vi "DATA MONITOR .vi"() -> ()   [LabVIEW 2018]
uses:
  <vilib>/Utility/miscctls.llb/LVRectTypeDef.ctl
panel:
  out "Date":string
  out "Year":string
  in  "Offset 7":u16 caption="Gain" max=100 format="%.0f "
  in  "Gain 7":u16 caption="Gain" max=100 format="%.0f "
  in  "Offset 5":u16 caption="Gain" max=100 format="%.0f "
  in  "Gain 5":u16 caption="Gain" max=100 format="%.0f "
  in  "Offset 6":u16 caption="Gain" max=100 format="%.0f "
  in  "Gain 6":u16 caption="Gain" max=100 format="%.0f "
  in  "Offset 3":u16 caption="Gain" max=100 format="%.0f "
  in  "Gain 3":u16 caption="Gain" max=100 format="%.0f "
  in  "Offset 4":u16 caption="Gain" max=100 format="%.0f "
  in  "Gain 4":u16 caption="Gain" max=100 format="%.0f "
  in  "Offset 1":u16 caption="Gain" max=100 format="%.0f "
  in  "Gain  1":u16 caption="Gain" max=100 format="%.0f "
  in  "Offset 2":u16 caption="Gain" max=100 format="%.0f "
  in  "Gain  2":u16 caption="Gain" max=100 format="%.0f "
  in  "Safety Limits":bool
  out "Dynamometer Torque N-m 8":dbl(knob) caption="Basement_T" scale=0.0..100.0
  out "Temperature PID":bool
  in  "Temperature":dbl(slide) scale=0.0..10.0
  out "Eng Rpm 2":dbl(knob) caption="Power" scale=0.0..10000.0
  out "Eng Rpm":dbl(knob) caption="Torque Summary" scale=0.0..10000.0
  out "Dynorpm":dbl(knob) caption="Speed Summary" scale=0.0..8000.0
  out "Dynamometer Torque N-m 7":dbl(knob) caption="Coolant_Outlet_T" scale=0.0..100.0
  out "Dynamometer Torque N-m 6":dbl(knob) caption="Coolant_Inlet_T" scale=0.0..100.0
  out "Dynamometer Torque N-m 5":dbl(knob) caption="Exhaust_T" scale=0.0..100.0
  out "Dynamometer Torque N-m 4":dbl(knob) caption="Oil_T" scale=0.0..100.0
  out "Dynamometer Torque N-m 3":dbl(knob) caption="Intercooler_Out_T" scale=0.0..100.0
  out "Dynamometer Torque N-m 2":dbl(knob) caption="Intercooler_In_T" scale=0.0..100.0
  in  "Reset":bool
  out "Alarms & Status":string
  in  "Tab Control":enum32{"Pressure  parameter", "Graph"}(tab)
  out "Ambient Temp. 2":dbl(slide) caption="Intercooler-In_P" scale=0.0..200.0
  out "Spark plug Temp":dbl(slide) caption="Coolant-Out_P" scale=0.0..200.0
  out "Oil Temp.":dbl(slide) caption="Coolant-In_P" scale=0.0..120.0
  out "Cylinder Block Temp.":dbl(slide) caption="Exhaust_P" scale=0.0..120.0
  out "ExhaustTemp.":dbl(slide) caption="Oil_P" scale=0.0..200.0
  out "Ambient Temp.":dbl(slide) caption="Intercooler-Out_P" scale=0.0..200.0
  out "T1":dbl(slide) caption="Misc_P" scale=0.0..100.0
  out "Chart 2":i32[](graph)
  out "eng model":string caption="Engine Model"
  out "eng type":string caption="Engine Type"
  out "NI cRIO Comm.":bool
  out "Test Cycle":dbl format="%<%H:%M:%S>t"
  in  "test stop":bool
  in  "start":bool
  in  "Home Button":bool
  # "ONLINE DATA"
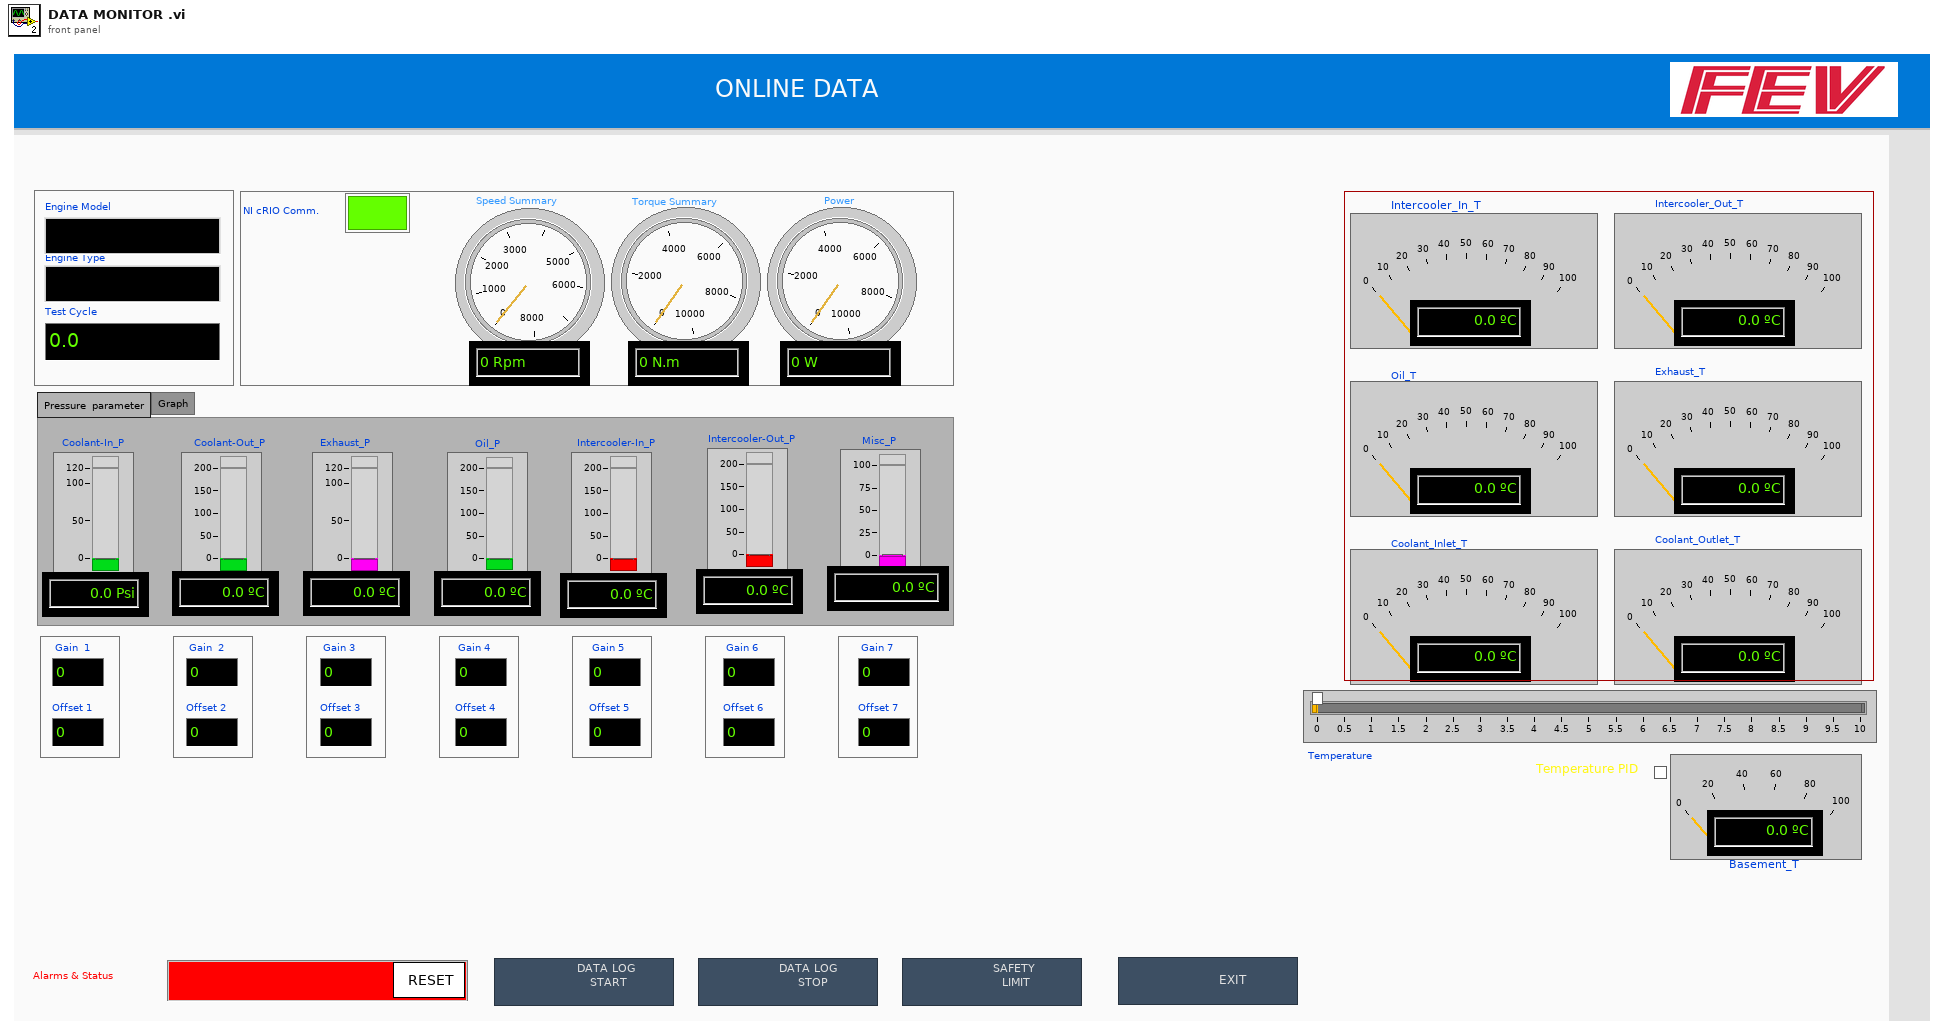
[diagram p1: front panel]
types:
  T1 = enum32{"Invalid", "Standard", "Closed", "Hidden", "Minimized", "Maximized"}
  T2 = enum32{"invalid app kind", "Development System", "Run Time System", "Student Edition", "Embedded LabVIEW", "Evaluation", "Custom"}
  T3 = typedef "LVRectTypeDef.ctl" = cluster{"Left":i16, "Top":i16, "Right":i16, "Bottom":i16}
  T4 = cluster{"Core":cluster{"Current VI Reference":refnum<vi>, "Close Panel on Exit?":bool}, "Your Boolean data":bool, "Your string data":string}
  T5 = cluster{"Current VI Reference":refnum<vi>, "Close Panel on Exit?":bool}
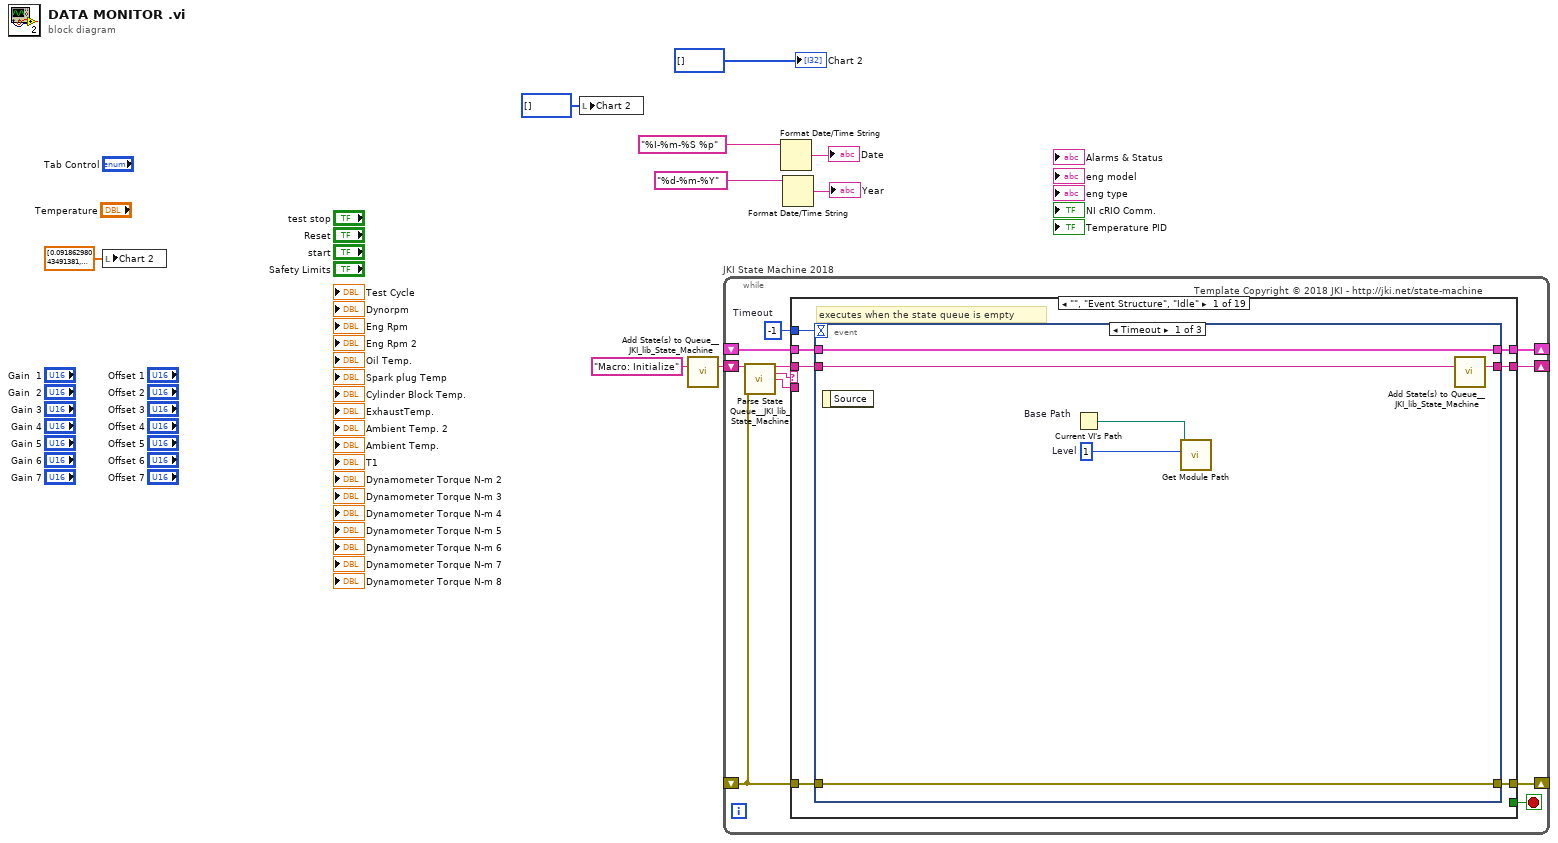
[diagram p0: block diagram]
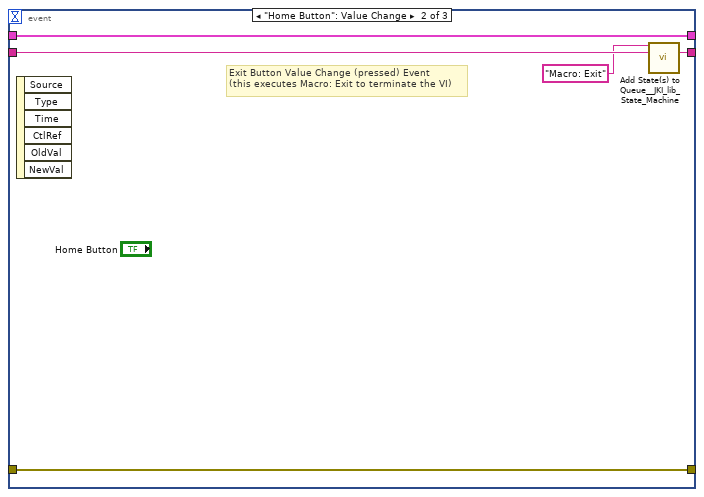
[diagram p2: hidden frame]
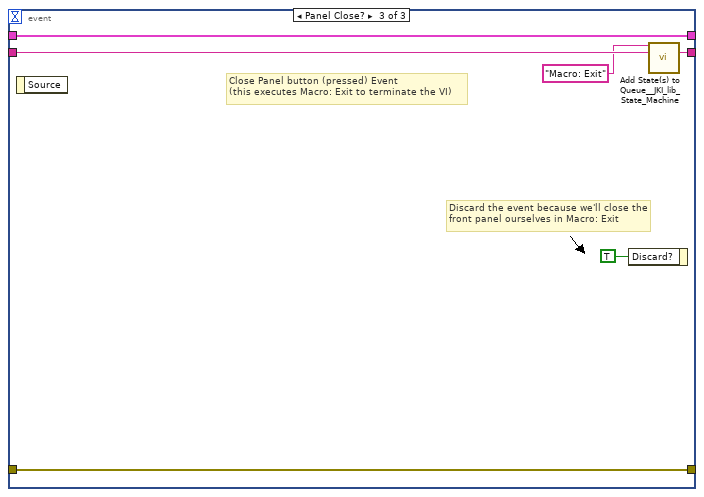
[diagram p3: hidden frame]
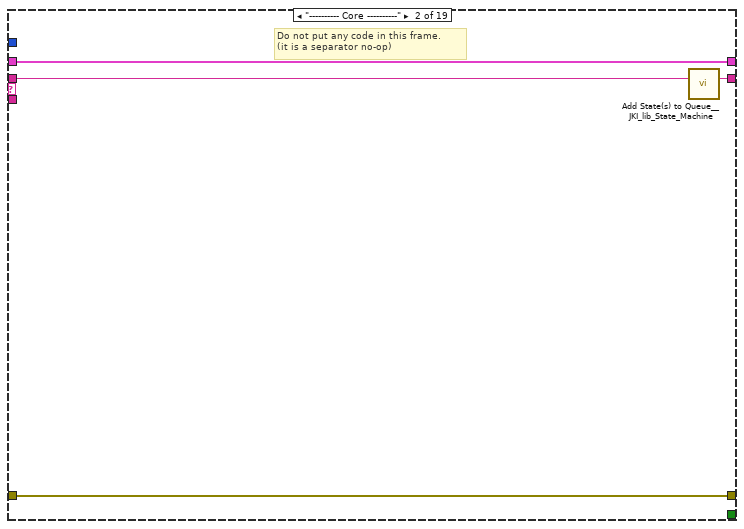
[diagram p4: hidden frame]
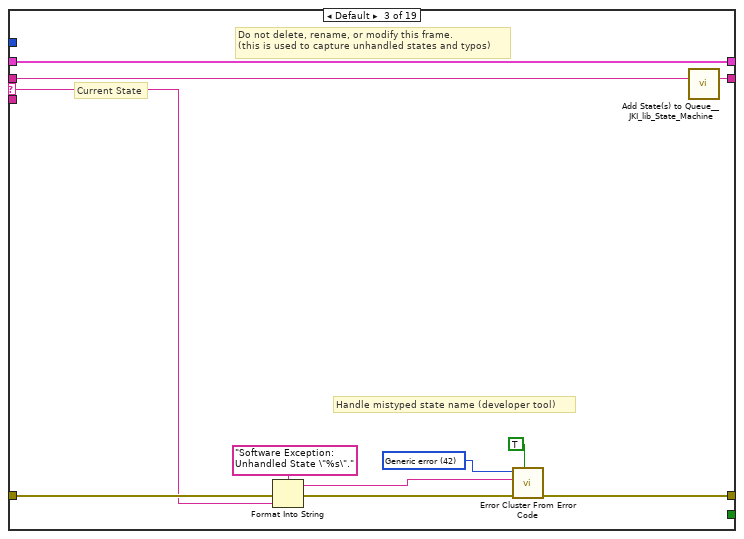
[diagram p5: hidden frame]
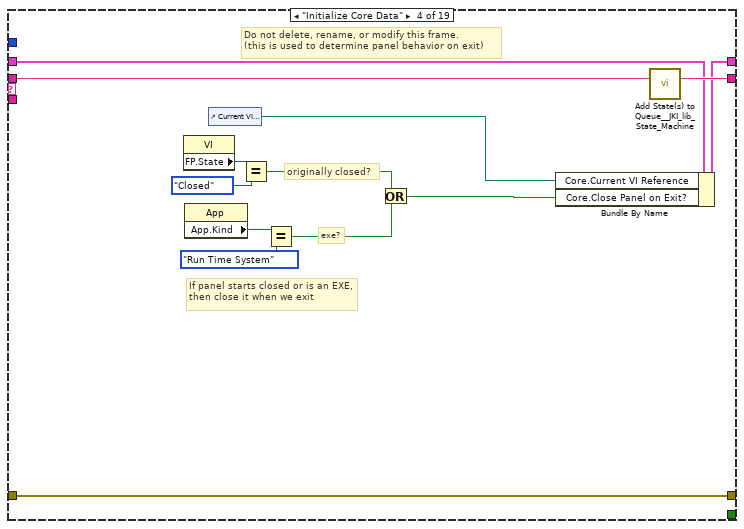
[diagram p6: hidden frame]
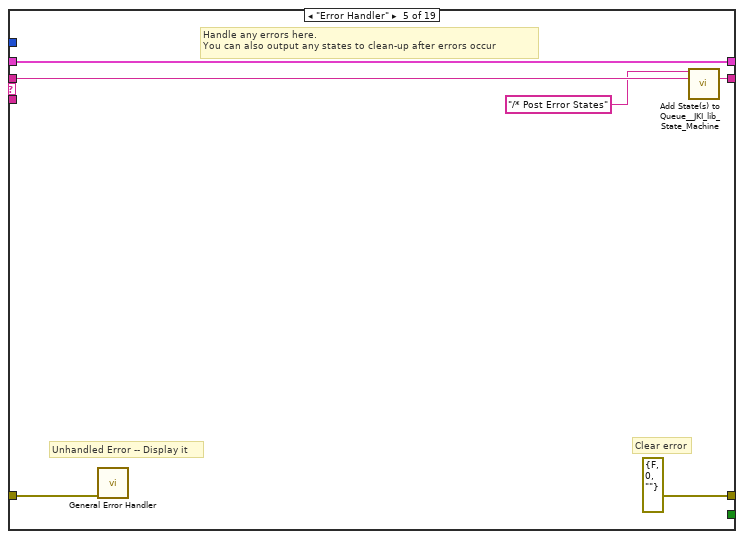
[diagram p7: hidden frame]
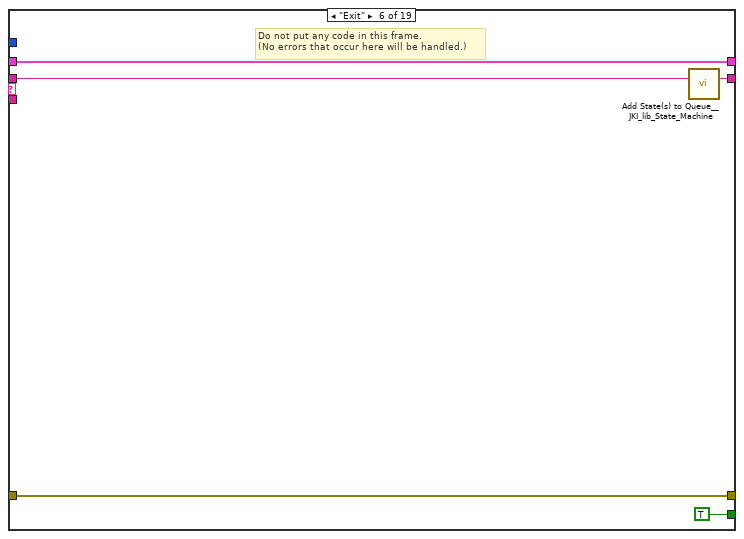
[diagram p8: hidden frame]
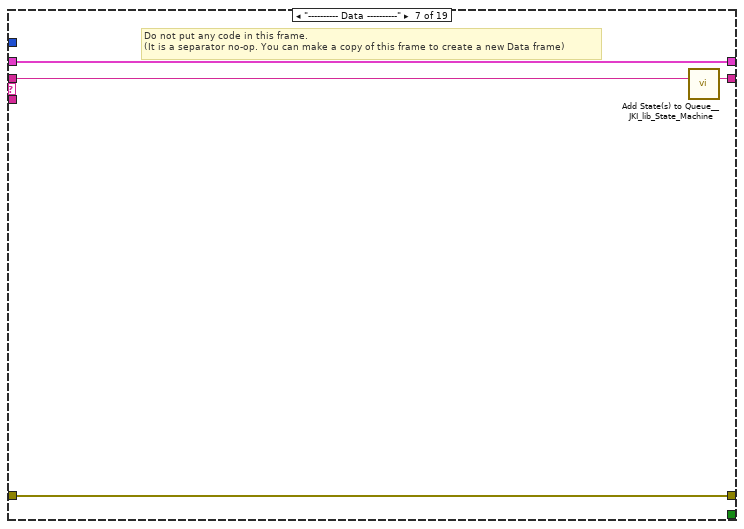
[diagram p9: hidden frame]
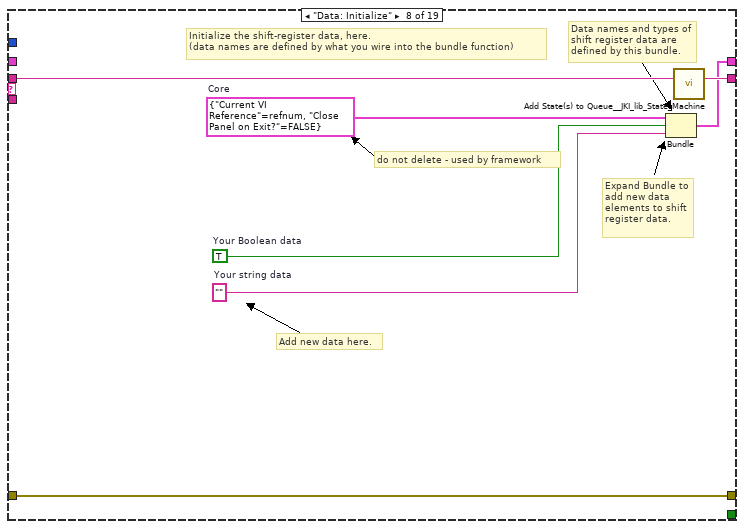
[diagram p10: hidden frame]
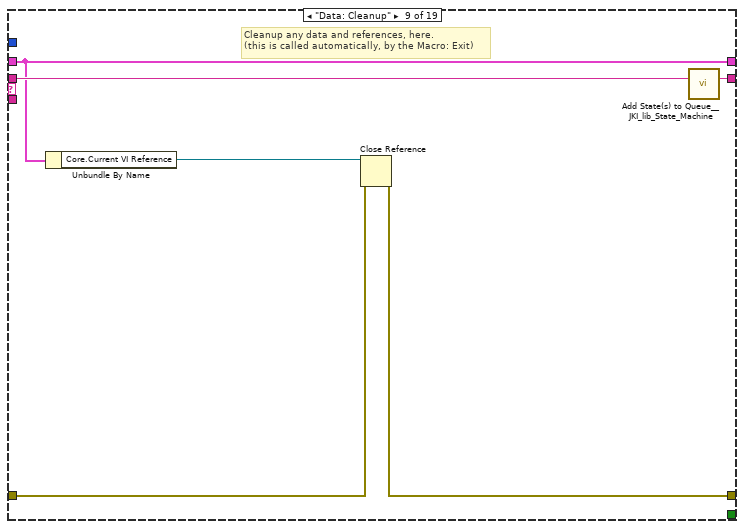
[diagram p11: hidden frame]
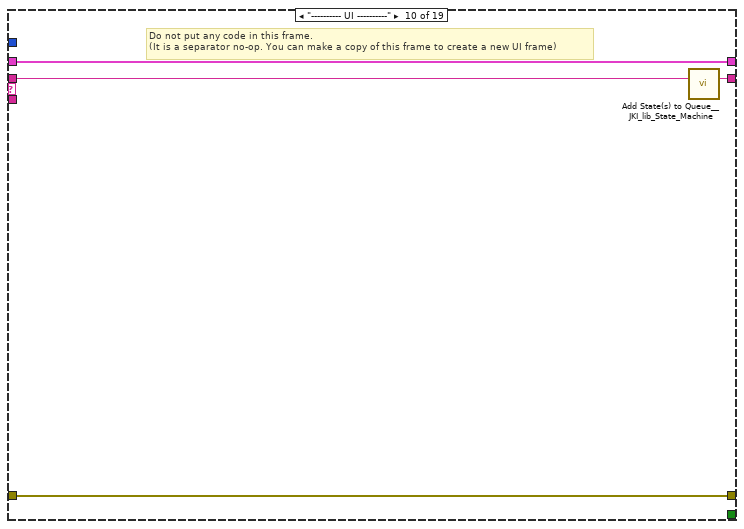
[diagram p12: hidden frame]
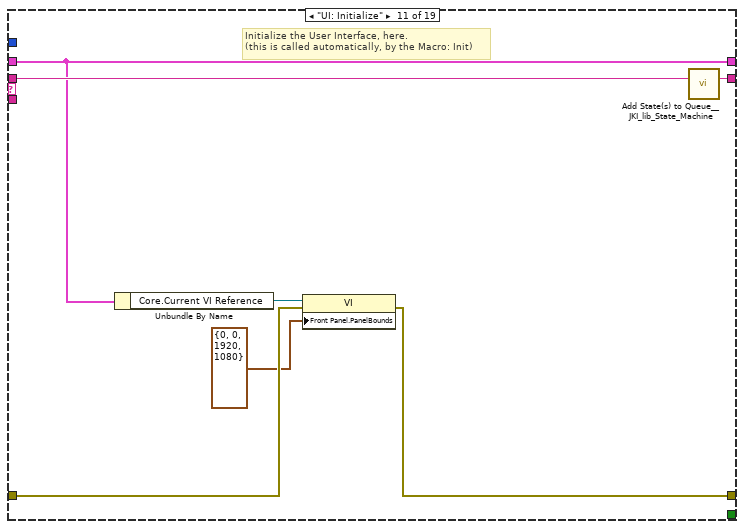
[diagram p13: hidden frame]
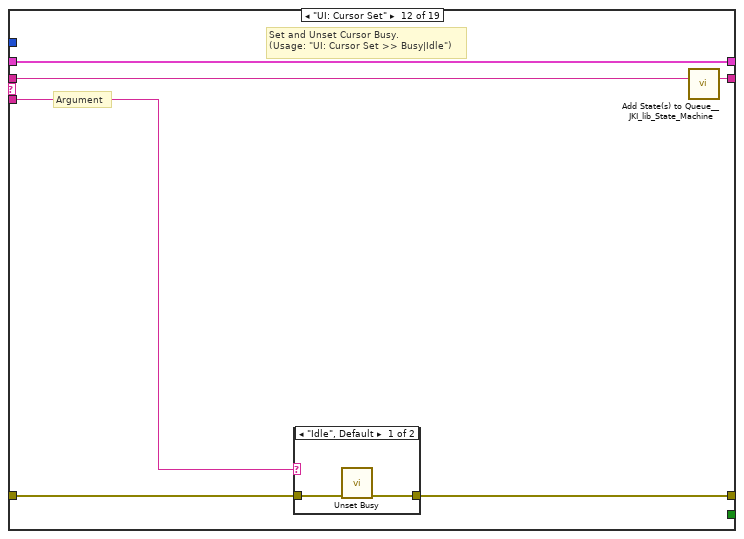
[diagram p14: hidden frame]
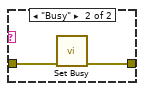
[diagram p15: hidden frame]
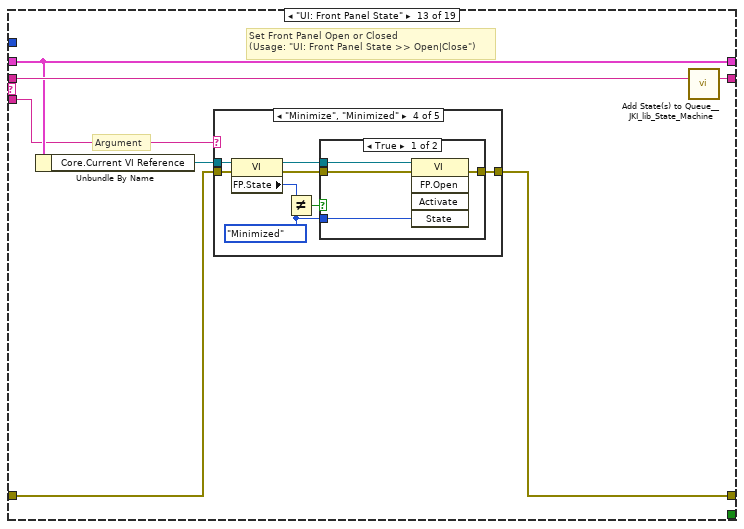
[diagram p16: hidden frame]
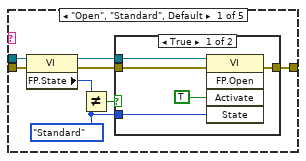
[diagram p17: hidden frame]
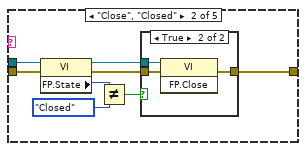
[diagram p19: hidden frame]
diagram:
  n1 = local write "Chart 2"(dbl[] [0.09186298043491381, 5.091862980434914, 0.09186298043491381] ("Chart 2")) -> ()
  n2 = local write "Chart 2"(i32[] [] ("Chart 2")) -> ()
  n3 = call <vilib>:"Add State(s) to Queue__JKI_lib_State_Machine.vi"("State(s) in (\"\")"="Macro: Initialize") -> ("States Out"=w2:string)  [unwired: 14 in]
  n4 = while "JKI State Machine 2018" {
    shift-right: [w13] -> _
    shift-left: _ -> [w12]
    shift-right: [w16] -> _
    shift-left: _ -> [w10]
    shift-right: [w15] -> _
    shift-left: w2 -> [w17]
    stop <- w14 stop-if-true
    w11 = -1  # Timeout
    # "Template Copyright © 2018 JKI - http://jki.net/state-machine"
    n5 = call <vilib>:"Parse State Queue__JKI_lib_State_Machine.vi"("State Queue"=w17, "Error In (no error)"=w10) -> ("Remaining States"=w19:string, "Current State"=w20:string, "Arguments"=w18:string)  [unwired: 11 in]
    n6 = case shown="\"\", \"Event Structure\", \"Idle\"" w20 {
      selector: w20 -> [_ _ w49 _ _ _ _ _ _ _ _ _ _ _ _ _ _ _ _]
      tunnel: w19 -> [w27 w48 w53 w72 w78 w83 w87 w94 w100 w104 w111 w117 w128 w197 w202 w212 w216 w220 w224]
      tunnel: w18 -> [_ _ _ _ _ _ _ _ _ _ _ w112 w122 _ _ _ _ _ _]
      tunnel: w12 -> [w25 w45 w51 w65 w75 w81 w84 _ w95 w101 w109 w115 w124 w194 w199 w209 w213 w217 w221]
      tunnel: [w24 w46 w55 w69 errorcluster {"status"=FALSE, "code"=0, "source"=""} ("error out") w80 w85 w91 w96 w102 w106 w113 w125 w195 w200 w210 w214 w218 w222] -> w16
      tunnel: w10 -> [w23 w46 w54 w69 w74 w80 w85 w91 w97 w102 w107 w114 w126 w195 w200 w210 w214 w218 w222]
      tunnel: [w26 w47 w52 w71 w77 w82 w86 w93 w99 w103 w110 w116 w127 w196 w201 w211 w215 w219 w223] -> w15
      tunnel: [_ _ _ _ _ TRUE _ _ _ _ _ _ _ _ _ _ _ _ _] -> w14
      tunnel: [w22 w45 w51 w70 w75 w81 w84 w92 w95 w101 w109 w115 w124 w194 w199 w209 w213 w217 w221] -> w13
      tunnel: w11 -> [w21 _ _ _ _ _ _ _ _ _ _ _ _ _ _ _ _ _ _]
      frame "", "Event Structure", "Idle" {
        # "executes when the state queue is empty"
        n7 = event shown="[0] Timeout" {
          selector: _ -> [_ _ _]
          dyn-events: _ -> [_ _ _]
          timeout: w21 -> [_ _ _]
          tunnel: w27 -> [w33 w38 w44]
          tunnel: [w32 w37 w43] -> w26
          tunnel: w25 -> [w30 w35 w41]
          tunnel: [w31 w36 w42] -> w24
          tunnel: w23 -> [w31 w36 w42]
          tunnel: [w30 w35 w41] -> w22
          event Timeout {
            w28 = 1  # Level
            n8 = event-data() -> ()  [unwired: 1 in, 1 out]
            n9 = Current VI's Path "Base Path"() -> (path=w29:path)
            n10 = call "Get Module Path.vi"("Level"=w28, "path"=w29) -> ()  [unwired: 8 in, 2 out]
            n11 = call <vilib>:"Add State(s) to Queue__JKI_lib_State_Machine.vi"("State(s) in (\"\")"=w33) -> ("States Out"=w32:string)  [unwired: 14 in]
          }
          event "Home Button": Value Change {
            # "Exit Button Value Change (pressed) Event\n(this executes Macro: Exit to terminate the VI)"
            n12 = event-data() -> ()  [unwired: 1 in, 6 out]
            n13 = call <vilib>:"Add State(s) to Queue__JKI_lib_State_Machine.vi"("State(s) in Front (\"\")"="Macro: Exit", "State(s) in (\"\")"=w38) -> ("States Out"=w37:string)  [unwired: 13 in]
          }
          event Panel Close? {
            # "Discard the event because we'll close the front panel ourselves in Macro: Exit"
            # "Close Panel button (pressed) Event\n(this executes Macro: Exit to terminate the VI)"
            n14 = event-data() -> ()  [unwired: 1 in, 1 out]
            n15 = event-data("Discard?"=TRUE) -> ()  [unwired: 1 in, 1 out]
            n16 = call <vilib>:"Add State(s) to Queue__JKI_lib_State_Machine.vi"("State(s) in Front (\"\")"="Macro: Exit", "State(s) in (\"\")"=w44) -> ("States Out"=w43:string)  [unwired: 13 in]
          }
        }
      }
      frame "---------- Core ----------" {
        # "Do not put any code in this frame.\n(it is a separator no-op)"
        n17 = call <vilib>:"Add State(s) to Queue__JKI_lib_State_Machine.vi"("State(s) in (\"\")"=w48) -> ("States Out"=w47:string)  [unwired: 14 in]
      }
      frame Default {
        w58 = 42 items=["No error", "Argument error", "Memory is full", "Out of zone", "End of file", "File already open", "Generic file I/O error", "File not found", "File permission error", "Disk is full", "Duplicate path", "Too many files open", "System feature not enabled", "Resource file not found", "Cannot add resource", "Resource not found", "Image not found", "Image memory error", "Pen does not exist", "Config type invalid", "Config token not found", "Config parse error", "Config memory error", "Bad external code format", "Bad external code offset", "External code not present", "Null window", "Destroy window error", "Null menu", "Print aborted", "Bad print record", "Print driver error", "Windows error during printing", "Memory error during printing", "Print dialog error", "Generic print error", "Invalid device refnum", "Device not found", "Device parameter error", "Device unit error", "Cannot open device", "Device call aborted", "Generic error", "Cancelled by user", "Object ID too low", "Object ID too high", "Object not in heap", "Unknown heap", "Unknown object (invalid DefProc)", "Unknown object (DefProc not in table)", "Message out of range", "Invalid (null) method", "Unknown message", "Manager call not supported", "Bad address", "Network operation in progress", "Network operation timed out", "Connection is busy", "Network attribute not supported", "Network error", "Address in use", "System out of memory", "Connection aborted", "Connection refused", "Not connected", "Already connected", "Connection closed", "Initialization error (interapplication manager)", "Bad occurrence", "Wait on unbound occurrence handler", "Occurrence queue overflow", "Datalog type conflict", "Unused", "Unrecognized type (interapplication manager)", "Memory corrupt", "Failed to make temporary DLL", "Old CIN version", "Drag socket not found", "Failed to load drop-object", "Failed to register OLE object", "Failed to release OLE object", "Format specifier type mismatch", "Unknown format specifier", "Too few format specifiers", "Too many format specifiers", "Scan failed", "Newer CIN version", "Error converting to variant", "Runtime menu error", "Password tampered", "Variant attribute not found", "Incompatible variant data type", "Event data is not available", "Event Store is not present", "Occurrence is not found", "Event Queue is not created", "Event info is not available", "Refnum passed is NULL", "Error retrieving Class GUID", "Error retrieving CoClass GUID", "Error retrieving TypeLib GUID.", "Bad built application magic bytes.", "Specific driver is different from the specific driver associated with the Logical Name.", "There is no session opened to the class driver.", "Max Error", "MAX - Error with config objects", "MAX - Error loading configuration", "MAX - Group not supported"]
        # "Current State"
        # "Do not delete, rename, or modify this frame.\n(this is used to capture unhandled states and typos)"
        # "Handle mistyped state name (developer tool)"
        n18 = Format Into String(format string="Software Exception: Unhandled State \"%s\"." ("message"), error in=w54, w49) -> (resulting string=w57:string, error out=w56:errorcluster)  [unwired: 1 in]
        n19 = call <vilib>:"Error Cluster From Error Code.vi"("show call chain? (False)"=TRUE, "error in (no error)"=w56, "error message (\"\")"=w57, "error code (0)"=w58) -> ("error out"=w55:errorcluster)  [unwired: 5 in]
        n20 = call <vilib>:"Add State(s) to Queue__JKI_lib_State_Machine.vi"("State(s) in (\"\")"=w53) -> ("States Out"=w52:string)  [unwired: 14 in]
      }
      frame "Initialize Core Data" {
        # "Do not delete, rename, or modify this frame.\n(this is used to determine panel behavior on exit)"
        # "originally closed?"
        # "exe?"
        # "If panel starts closed or is an EXE, then close it when we exit"
        n21 = property class="VI"() -> ("FP.State"=w62:T1)  [unwired: 2 in, 2 out]
        n22 = property class="App"() -> ("App.Kind"=w68:T2)  [unwired: 2 in, 2 out]
        n23 = control-ref of="Current VI Reference"() -> (w63:refnum<vi>)
        n24 = Equal?(x=w62, y=T1."Closed" ("Front Panel Window:State")) -> (x = y?=w60:bool)
        n25 = Equal?(x=w68, y=T2."Run Time System" ("Application:Kind")) -> (x = y?=w66:bool)
        n26 = Or(x=w60, y=w66) -> (x .or. y?=w64:bool)
        n27 = Bundle By Name(cluster=w65, "Core.Current VI Reference"=w63, "Core.Close Panel on Exit?"=w64) -> (w70:T4)
        n28 = call <vilib>:"Add State(s) to Queue__JKI_lib_State_Machine.vi"("State(s) in (\"\")"=w72) -> ("States Out"=w71:string)  [unwired: 14 in]
      }
      frame "Error Handler" {
        # "Unhandled Error -- Display it"
        # "Handle any errors here.\nYou can also output any states to clean-up after errors occur"
        # "Clear error"
        n29 = call <vilib>:"General Error Handler.vi"("error in (no error)"=w74) -> ()  [unwired: 10 in, 5 out]
        n30 = call <vilib>:"Add State(s) to Queue__JKI_lib_State_Machine.vi"("State(s) in Front (\"\")"="/* Post Error States", "State(s) in (\"\")"=w78) -> ("States Out"=w77:string)  [unwired: 13 in]
      }
      frame "Exit" {
        # "Do not put any code in this frame.\n(No errors that occur here will be handled.)"
        n31 = call <vilib>:"Add State(s) to Queue__JKI_lib_State_Machine.vi"("State(s) in (\"\")"=w83) -> ("States Out"=w82:string)  [unwired: 14 in]
      }
      frame "---------- Data ----------" {
        # "Do not put any code in this frame.\n(It is a separator no-op. You can make a copy of this frame to create a new Data frame)"
        n32 = call <vilib>:"Add State(s) to Queue__JKI_lib_State_Machine.vi"("State(s) in (\"\")"=w87) -> ("States Out"=w86:string)  [unwired: 14 in]
      }
      frame "Data: Initialize" {
        w88 = T5 {"Current VI Reference"=refnum, "Close Panel on Exit?"=FALSE}  # Core
        w90 = TRUE  # Your Boolean data
        w89 = ""  # Your string data
        # "do not delete - used by framework"
        # "Expand Bundle to add new data elements to shift register data."
        # "Add new data here."
        # "Data names and types of shift register data are defined by this bundle."
        # "Initialize the shift-register data, here.\n(data names are defined by what you wire into the bundle function)"
        n33 = Bundle("Core"=w88, "Your Boolean data"=w90, "Your string data"=w89) -> (w92:T4)  [unwired: 1 in]
        n34 = call <vilib>:"Add State(s) to Queue__JKI_lib_State_Machine.vi"("State(s) in (\"\")"=w94) -> ("States Out"=w93:string)  [unwired: 14 in]
      }
      frame "Data: Cleanup" {
        # "Cleanup any data and references, here.\n(this is called automatically, by the Macro: Exit)"
        n35 = Unbundle By Name(w95) -> ("Core.Current VI Reference"=w98:refnum<vi>)
        n36 = Close Reference(reference=w98, error in (no error)=w97) -> (error out=w96:errorcluster)
        n37 = call <vilib>:"Add State(s) to Queue__JKI_lib_State_Machine.vi"("State(s) in (\"\")"=w100) -> ("States Out"=w99:string)  [unwired: 14 in]
      }
      frame "---------- UI ----------" {
        # "Do not put any code in this frame.\n(It is a separator no-op. You can make a copy of this frame to create a new UI frame)"
        n38 = call <vilib>:"Add State(s) to Queue__JKI_lib_State_Machine.vi"("State(s) in (\"\")"=w104) -> ("States Out"=w103:string)  [unwired: 14 in]
      }
      frame "UI: Initialize" {
        # "Initialize the User Interface, here.\n(this is called automatically, by the Macro: Init)"
        n39 = Unbundle By Name(w109) -> ("Core.Current VI Reference"=w108:refnum<vi>)
        n40 = property class="VI"(reference=w108, error in=w107, "Front Panel.PanelBounds"=T3 {"Left"=0, "Top"=0, "Right"=1920, "Bottom"=1080} ("Front Panel Window:Panel Bounds")) -> (error out=w106:errorcluster)  [unwired: 1 out]
        n41 = call <vilib>:"Add State(s) to Queue__JKI_lib_State_Machine.vi"("State(s) in (\"\")"=w111) -> ("States Out"=w110:string)  [unwired: 14 in]
      }
      frame "UI: Cursor Set" {
        # "Argument"
        # "Set and Unset Cursor Busy.\n(Usage: \"UI: Cursor Set >> Busy|Idle\")"
        n42 = case shown="\"Idle\", Default" w112 {
          tunnel: w114 -> [w119 w121]
          tunnel: [w118 w120] -> w113
          frame "Idle", Default {
            n43 = call <vilib>:"Unset Busy.vi"("error in (no error)"=w119) -> ("error out"=w118:errorcluster)  [unwired: 10 in]
          }
          frame "Busy" {
            n44 = call <vilib>:"Set Busy.vi"("error in (no error)"=w121) -> ("error out"=w120:errorcluster)  [unwired: 9 in, 1 out]
          }
        }
        n45 = call <vilib>:"Add State(s) to Queue__JKI_lib_State_Machine.vi"("State(s) in (\"\")"=w117) -> ("States Out"=w116:string)  [unwired: 14 in]
      }
      frame "UI: Front Panel State" {
        # "Argument"
        # "Set Front Panel Open or Closed\n(Usage: \"UI: Front Panel State >> Open|Close\")"
        n46 = Unbundle By Name(w124) -> ("Core.Current VI Reference"=w123:refnum<vi>)
        n47 = case shown="\"Minimize\", \"Minimized\"" w122 {
          tunnel: w126 -> [w134 w149 w160 w173 w186]
          tunnel: [w136 w150 w162 w175 w188] -> w125
          tunnel: w123 -> [w135 w147 w161 w174 w187]
          frame "Open", "Standard", Default {
            w129 = T1."Standard" ("State")
            n48 = property class="VI"(reference=w135, error in=w134) -> (reference out=w132:refnum<vi>, error out=w133:errorcluster, "FP.State"=w131:T1)
            n49 = Not Equal?(x=w131, y=w129) -> (x != y?=w130:bool)
            n50 = case shown="True" w130 {
              tunnel: [w140 w142] -> w136
              tunnel: w133 -> [w139 w142]
              tunnel: w132 -> [w138 _]
              tunnel: w129 -> [w137 _]
              frame True {
                n51 = invoke class="VI" method="FP.Open"(reference=w138, error in=w139, "Activate"=TRUE, "State"=w137) -> (error out=w140:errorcluster)  [unwired: 1 in, 4 out]
              }
              frame False {
              }
            }
          }
          frame "Close", "Closed" {
            n52 = property class="VI"(reference=w147, error in=w149) -> (reference out=w146:refnum<vi>, error out=w148:errorcluster, "FP.State"=w144:T1)
            n53 = Not Equal?(x=w144, y=T1."Closed" ("Front Panel Window:State")) -> (x != y?=w143:bool)
            n54 = case shown="True" w143 {
              tunnel: [w151 w154] -> w150
              tunnel: w148 -> [w151 w153]
              tunnel: w146 -> [_ w152]
              frame False {
              }
              frame True {
                n55 = invoke class="VI" method="FP.Close"(reference=w152, error in=w153) -> (error out=w154:errorcluster)  [unwired: 1 in, 2 out]
              }
            }
          }
          frame "Hidden", "Hide" {
            w155 = T1."Hidden" ("State")
            n56 = property class="VI"(reference=w161, error in=w160) -> (reference out=w158:refnum<vi>, error out=w159:errorcluster, "FP.State"=w157:T1)
            n57 = Not Equal?(x=w157, y=w155) -> (x != y?=w156:bool)
            n58 = case shown="True" w156 {
              tunnel: [w166 w167] -> w162
              tunnel: w159 -> [w165 w167]
              tunnel: w158 -> [w164 _]
              tunnel: w155 -> [w163 _]
              frame True {
                n59 = invoke class="VI" method="FP.Open"(reference=w164, error in=w165, "State"=w163) -> (error out=w166:errorcluster)  [unwired: 2 in, 4 out]
              }
              frame False {
              }
            }
          }
          frame "Minimize", "Minimized" {
            w168 = T1."Minimized" ("State")
            n60 = property class="VI"(reference=w174, error in=w173) -> (reference out=w171:refnum<vi>, error out=w172:errorcluster, "FP.State"=w170:T1)
            n61 = Not Equal?(x=w170, y=w168) -> (x != y?=w169:bool)
            n62 = case shown="True" w169 {
              tunnel: [w179 w180] -> w175
              tunnel: w172 -> [w178 w180]
              tunnel: w171 -> [w177 _]
              tunnel: w168 -> [w176 _]
              frame True {
                n63 = invoke class="VI" method="FP.Open"(reference=w177, error in=w178, "State"=w176) -> (error out=w179:errorcluster)  [unwired: 2 in, 4 out]
              }
              frame False {
              }
            }
          }
          frame "Maximize", "Maximized" {
            w181 = T1."Maximized" ("State")
            n64 = property class="VI"(reference=w187, error in=w186) -> (reference out=w184:refnum<vi>, error out=w185:errorcluster, "FP.State"=w183:T1)
            n65 = Not Equal?(x=w183, y=w181) -> (x != y?=w182:bool)
            n66 = case shown="True" w182 {
              tunnel: [w192 w193] -> w188
              tunnel: w185 -> [w191 w193]
              tunnel: w184 -> [w190 _]
              tunnel: w181 -> [w189 _]
              frame True {
                n67 = invoke class="VI" method="FP.Open"(reference=w190, error in=w191, "State"=w189) -> (error out=w192:errorcluster)  [unwired: 2 in, 4 out]
              }
              frame False {
              }
            }
          }
        }
        n68 = call <vilib>:"Add State(s) to Queue__JKI_lib_State_Machine.vi"("State(s) in (\"\")"=w128) -> ("States Out"=w127:string)  [unwired: 14 in]
      }
      frame "---------- Macro ----------" {
        # "Do not put any code in this frame.\n(It is a separator no-op. You can make a copy of this frame to create a new Macro frame)"
        n69 = call <vilib>:"Add State(s) to Queue__JKI_lib_State_Machine.vi"("State(s) in (\"\")"=w197) -> ("States Out"=w196:string)  [unwired: 14 in]
      }
      frame "Macro: Initialize" {
        w198 = "Data: Initialize\nInitialize Core Data\nUI: Initialize\nUI: Front Panel State >> Open"  # Data: Initialize Initialize Core Data UI: Initialize UI: Front Panel State >> Open
        # "Initialization Macro\n(This is called once, when the VI starts)"
        n70 = call <vilib>:"Add State(s) to Queue__JKI_lib_State_Machine.vi"("State(s) in Front (\"\")"=w198, "State(s) in (\"\")"=w202) -> ("States Out"=w201:string)  [unwired: 13 in]
      }
      frame "Macro: Exit" {
        # "Exit Macro\n(This is called once, when the VI exits)"
        n71 = Unbundle By Name(w209) -> ("Core.Close Panel on Exit?"=w208:bool)
        n72 = Select(t="UI: Front Panel State >> Close", s=w208, f="") -> (s? t:f=w205:string)
        n73 = call <vilib>:"Add State(s) to Queue__JKI_lib_State_Machine.vi"("State(s) in (\"\")"=w205, "State(s) at Back (\"\")"="Data: Cleanup\nExit") -> ("States Out"=w203:string)  [unwired: 13 in]
        n74 = call <vilib>:"Add State(s) to Queue__JKI_lib_State_Machine.vi"("State(s) in Front (\"\")"=w203, "State(s) in (\"\")"=w212) -> ("States Out"=w211:string)  [unwired: 13 in]
      }
      frame "---------- New Category ----------" {
        # "Template Separator\n(You can make a copy of, or modify, this frame)"
        n75 = call <vilib>:"Add State(s) to Queue__JKI_lib_State_Machine.vi"("State(s) in (\"\")"=w216) -> ("States Out"=w215:string)  [unwired: 14 in]
      }
      frame "New Category: 1" {
        # "Your code here.\n(You can make a copy of, or modify, this frame)"
        n76 = call <vilib>:"Add State(s) to Queue__JKI_lib_State_Machine.vi"("State(s) in (\"\")"=w220) -> ("States Out"=w219:string)  [unwired: 14 in]
      }
      frame "New Category: 2" {
        # "Your code here.\n(You can make a copy of, or modify, this frame)"
        n77 = call <vilib>:"Add State(s) to Queue__JKI_lib_State_Machine.vi"("State(s) in (\"\")"=w224) -> ("States Out"=w223:string)  [unwired: 14 in]
      }
    }
  }
  n78 = Format Date/Time String(time format string (%c)="%I-%m-%S %p") -> (date/time string=→"Date":string)  [unwired: 2 in]
  n79 = Format Date/Time String(time format string (%c)="%d-%m-%Y") -> (date/time string=→"Year":string)  [unwired: 2 in]
  "Chart 2" <- i32[] [] ("Chart 2")
